vi "HW_QX_Refresh Tree Device Info.vi"(8 "error in":errorcluster caption="错误输入", 10 "QXModuInfo":T1[](array[typedef]), 11 "Ref.Tree Ref":refnum<vi>) -> (0 "error out":errorcluster caption="错误输出")   [LabVIEW 2016]
uses:
  QX Module Info.ctl
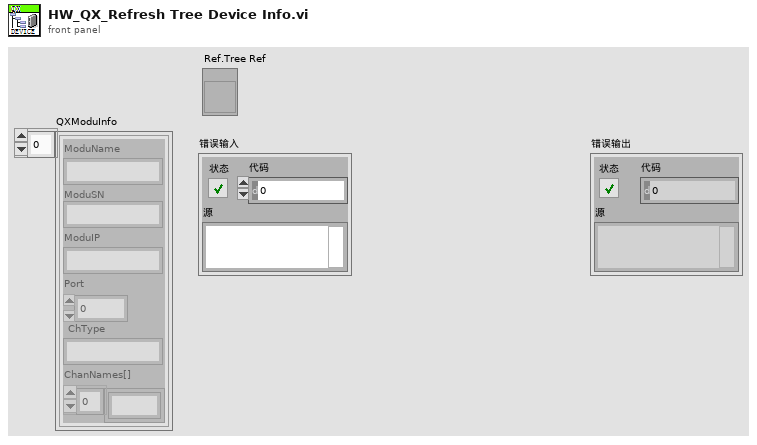
[diagram p1: front panel]
types:
  T1 = typedef "QX Module Info.ctl" = cluster{"ModuName":string, "ModuSN":string, "ModuIP":string, "Port":i32, "ChType":string, "ChanNames[]":string[]}
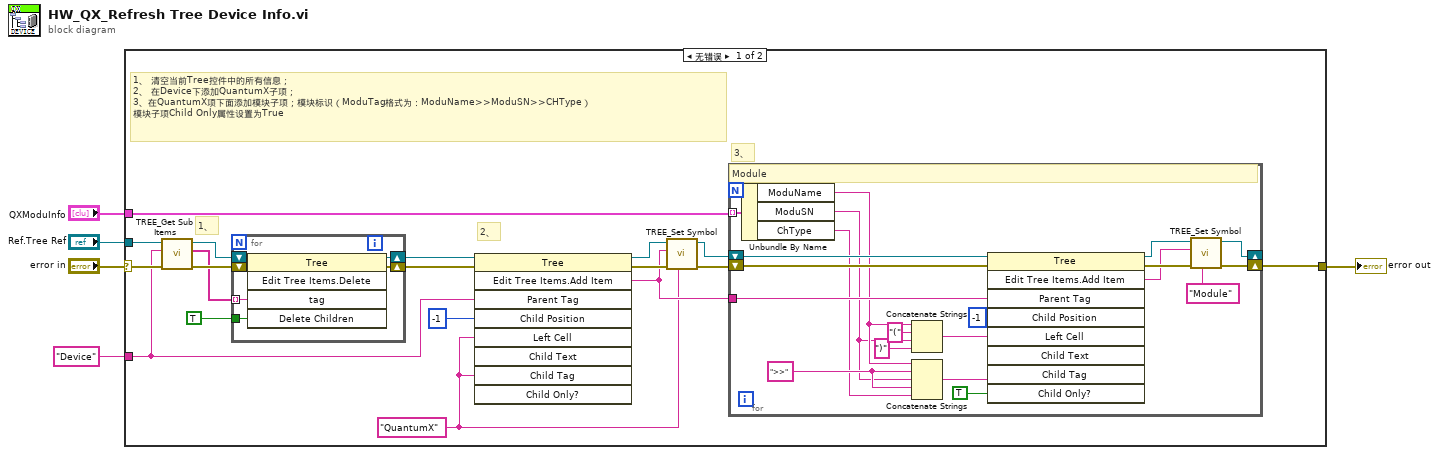
[diagram p0: block diagram]
diagram:
  n1 = case shown="无错误" "error in" {
    selector: "error in" -> [w19 w50]
    tunnel: [w23 w50] -> w4
    tunnel: "Ref.Tree Ref" -> [w17 _]
    tunnel: "Device" ("PicName") -> [w16 _]
    tunnel: "QXModuInfo" -> [w6 _]
    frame No Error {
      w7 = "QuantumX" ("Left Cell String")
      # "3、"
      # "2、"
      # "1、"
      # "1、 清空当前Tree控件中的所有信息；\n2、 在Device下添加QuantumX子项；\n3、在QuantumX项下面添加模块子项；模块标识（ModuTag格式为：ModuName>>ModuSN>>CHType）\n模块子项Child Only属性设置为True"
      n2 = call "TREE_Get Sub Items.vi"("error in"=w19, "Par Tag"=w16, "TreeRef"=w17) -> ("error out"=w18:errorcluster, "Tags"=w14:string[], "TreeRef"=w15:refnum<vi>)  [unwired: 5 in, 1 out]
      n3 = for {
        tunnel: TRUE ("删除子项？") -> [w47]
        shift-right: [w48] -> w21
        shift-left: w18 -> [w46]
        shift-right: [w49] -> w22
        shift-left: w15 -> [w45]
        tunnel: w14 -> [w44] mode=indexing
        n4 = invoke class="Tree" method="Edit Tree Items.Delete"(reference=w45, error in=w46, "tag"=w44, "Delete Children"=w47) -> (reference out=w49:refnum<vi>, error out=w48:errorcluster)  [unwired: 1 in, 3 out]
      }
      n5 = invoke class="Tree" method="Edit Tree Items.Add Item"(reference=w22, error in=w21, "Parent Tag"=w16, "Child Position"=-1 ("子项位置"), "Left Cell"=w7, "Child Tag"=w7) -> (reference out=w11:refnum<vi>, error out=w13:errorcluster, "Edit Tree Items:Add Item"=w9:string)  [unwired: 3 in, 6 out]
      n6 = call "TREE_Set Symbol.vi"("PicName"=w7, "error in"=w13, "Tag"=w9, "Tree Ref"=w11) -> ("error out"=w12:errorcluster, "Tree Ref"=w10:refnum<vi>)  [unwired: 6 in]
      n7 = for {
        shift-right: [w34] -> _
        shift-left: w10 -> [w41]
        shift-right: [w36] -> w23
        shift-left: w12 -> [w40]
        tunnel: w9 -> [w38]
        tunnel: w6 -> [w43] mode=indexing
        w29 = ">>" ("字符串")
        # "Module"
        n8 = Unbundle By Name(w43) -> ("ModuName"=w30:string, "ModuSN"=w26:string, "ChType"=w28:string)
        n9 = Concatenate Strings(w30, "(" ("string"), w26, ")" ("string")) -> (w27:string)
        n10 = Concatenate Strings(w30, w29, w26, w29, w28) -> (w42:string)
        n11 = invoke class="Tree" method="Edit Tree Items.Add Item"(reference=w41, error in=w40, "Parent Tag"=w38, "Child Position"=-1 ("子项位置"), "Left Cell"=w27, "Child Tag"=w42, "Child Only?"=TRUE ("仅作为子项？")) -> (reference out=w35:refnum<vi>, error out=w37:errorcluster, "Edit Tree Items:Add Item"=w33:string)  [unwired: 2 in, 6 out]
        n12 = call "TREE_Set Symbol.vi"("PicName"="Module", "error in"=w37, "Tag"=w33, "Tree Ref"=w35) -> ("error out"=w36:errorcluster, "Tree Ref"=w34:refnum<vi>)  [unwired: 6 in]
      }
    }
    frame Error {
    }
  }
  "error out" <- w4
